vi "SetNotifier.vi"(8 "error in (no error)":errorcluster, 10 "notifier":refnum<notifier>, 11 "ClassByRef in":refnum<class "ClassByRef.lvclass">) -> (0 "error out":errorcluster, 3 "ClassByRef out":refnum<class "ClassByRef.lvclass">)   [LabVIEW 2021, in "ClassUtilities.lvlib" / "ClassByRef.lvclass"]
uses:
  ClassByRef.lvclass
  ClassByRef.lvclass/ClassByRef.ctl
  6a7be9d6-cac5-4ac9-b7fd-da113b1d2d73.vi
  GetRef.vi
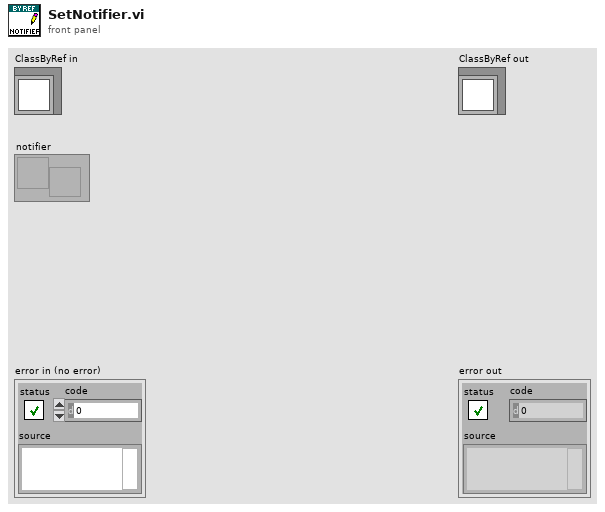
[diagram p1: front panel]
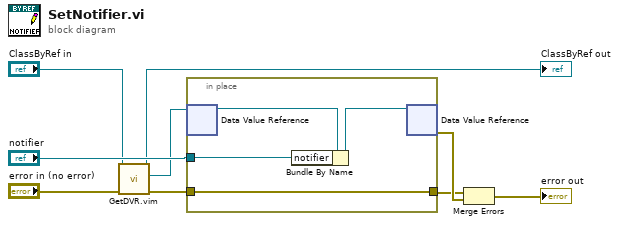
[diagram p0: block diagram]
diagram:
  n1 = call "GetDVR.vim"("error in (no error)"="error in (no error)", "ByRefClass in"="ClassByRef in") -> ("error out"=w4:errorcluster, "DVR"=w1:refnum<data-value>, "ByRefClass out"=→"ClassByRef out":refnum<class "ClassByRef.lvclass">)  [unwired: 7 in]
  n2 = in-place {
    in-place-border: w4 -> [w13]
    in-place-border: [w13] -> w8
    in-place-border: "notifier" -> [w10]
    n3 = in-place-dvr #1(w1) -> (w11:refnum<class "ClassByRef.lvclass">)  [unwired: 1 out]
    n4 = Bundle By Name(cluster=w11, "notifier"=w10) -> (w12:refnum<class "ClassByRef.lvclass">)
    n5 = in-place-dvr #1(w12) -> (w9:errorcluster)  [unwired: 1 out]
  }
  n6 = Merge Errors(w8, w9) -> (→"error out":errorcluster)
